vi "List Error Cluster Attributes.vi"(11 "error":errorcluster) -> (3 "attribute names":string[](array[string]))   [LabVIEW 2020, in "Multi Error Cluster.lvlib"]
doc: "Returns the names of all attributes stored in an error cluster. For a single cluster that stores multiple errors, this VI lists only the attribute names of the first error."
uses:
  <vilib>/MultiError/TokenizeJSON/Multi Error Cluster.lvlib
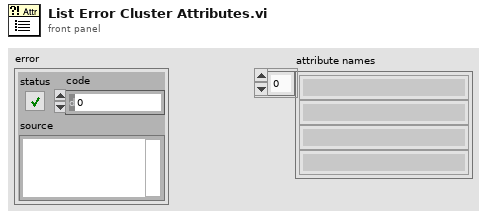
[diagram p1: front panel]
types:
  T1 = typedef "Multi Error Cluster.lvlib/JSON Object Descriptor.ctl" = cluster{"begin info":T2, "end info":T2, "begin Index":i32, "end Index":i32}
  T2 = typedef "Multi Error Cluster.lvlib/JSON Token Descriptor.ctl" = cluster{"match string":string, "raw token type":T3, "byte offset ":i32}
  T3 = typedef "Multi Error Cluster.lvlib/JSON Raw Token Values.ctl" = enum32{"{", "}", "[", "]", ",", ":", "\"", "number", "string", "true", "false", "null", "invalid"}
  T4 = typedef "Multi Error Cluster.lvlib/JSON Token Values.ctl" = enum32{"array begin", "array end", "object begin", "object end", "value", "invalid", "name"}
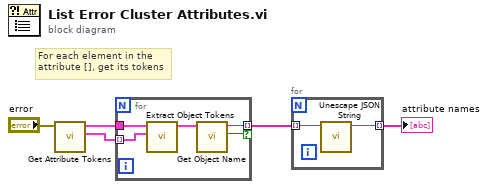
[diagram p0: block diagram]
diagram:
  # "For each element in the\nattribute [], get its tokens"
  n1 = call <vilib>:"Get Attribute Tokens.vi"("error"="error") -> ("array of JSON objects"=w3:T1[], "attribute tokens"=w5:cluster{"token type":T4, T2}[])  [unwired: 8 in, 1 out]
  n2 = for {
    tunnel: w5 -> [w7]
    tunnel: [w10] -> w2 mode=indexing if=w9
    tunnel: w3 -> [w8] mode=indexing
    n3 = call <vilib>:"Extract Object Tokens.vi"("JSON Object Descriptor"=w8, "attribute tokens"=w7) -> ("Extracted Tokens"=w6:cluster{"token type":T4, T2}[])  [unwired: 9 in]
    n4 = call <vilib>:"Get Object Name.vi"("Extracted Tokens"=w6) -> ("found"=w9:bool, "name"=w10:string)  [unwired: 9 in]
  }
  n5 = for {
    tunnel: w2 -> [w12] mode=indexing
    tunnel: [w11] -> w1 mode=indexing
    n6 = call <vilib>:"Unescape JSON String.vi"("escaped string"=w12) -> ("regular string"=w11:string)  [unwired: 10 in]
  }
  "attribute names" <- w1
